vi "Spartan HTTP Error Reply.vi"(2 "message":string, 3 "status code":i32) -> (0 "content":string, 1 "header":string)   [LabVIEW 2011]
uses:
  Addons/internet/http/config.llb/HTTP SRM.vi
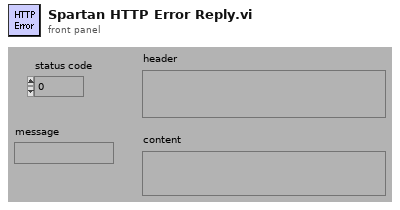
[diagram p1: front panel]
types:
  T1 = typedef "Keyed Array.ctl" = cluster{"keys":string[], "values":string[]}
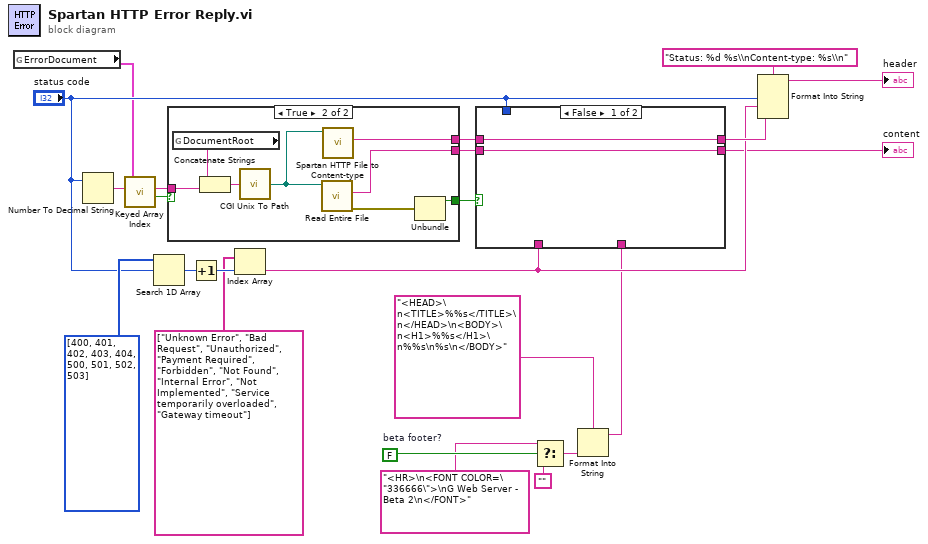
[diagram p0: block diagram]
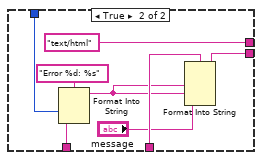
[diagram p2: hidden frame]
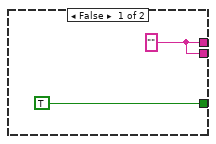
[diagram p3: hidden frame]
diagram:
  w5 = FALSE  # beta footer?
  n1 = global read "HTTP SRM.vi" "ErrorDocument"() -> (w1:T1)
  n2 = Number To Decimal String(number="status code") -> (decimal integer string=w18:string)  [unwired: 1 out]
  n3 = call "Keyed Array Index.vi"("key"=w18, "array in"=w1) -> ("valid key"=w17:bool, "value"=w16:string)  [unwired: 2 in, 2 out]
  n4 = Search 1D Array(1D array=i32[] [400, 401, 402, 403, 404, 500, 501, 502, 503], element="status code") -> (index of element=w22:i32)  [unwired: 1 out]
  n5 = case shown="True" w17 {
    tunnel: w16 -> [_ w31]
    tunnel: [TRUE ("status") w33] -> w15
    tunnel: [w24 w30] -> w14
    tunnel: [w24 w27] -> w13
    frame False {
      w24 = "" ("content type")
    }
    frame True {
      n6 = global read "HTTP SRM.vi" "DocumentRoot"() -> (w26:string)
      n7 = Concatenate Strings(w26, w31) -> (w32:string)
      n8 = call "CGI Unix To Path.vi"("unix path"=w32) -> ("platform path"=w29:path)  [unwired: 1 out]
      n9 = call "Read Entire File.vi"("path"=w29) -> ("error out"=w28:errorcluster, "data"=w27:string)  [unwired: 2 in, 7 out]
      n10 = call "Spartan HTTP File to Content-type.vi"("file path"=w29) -> ("content-type"=w30:string)  [unwired: 3 in, 7 out]
      n11 = Unbundle(w28) -> ("status"=w33:bool)  [unwired: 2 out]
    }
  }
  n12 = Increment(x=w22) -> (x+1=w23:i32)
  n13 = Index Array(array=string[] ["Unknown Error", "Bad Request", "Unauthorized", "Payment Required", "Forbidden", "Not Found", "Internal Error", "Not Implemented", "Service temporarily overloaded", "Gateway timeout"], index=w23) -> (element=w11:string)
  n14 = Select(t="<HR>\n<FONT COLOR=\"336666\">\nG Web Server - Beta 2\n</FONT>", s=w5, f="") -> (s? t:f=w3:string)
  n15 = Format Into String(format string="<HEAD>\n<TITLE>%%s</TITLE>\n</HEAD>\n<BODY>\n<H1>%%s</H1>\n%%s\n%s\n</BODY>", w3) -> (resulting string=w8:string)  [unwired: 2 in, 1 out]
  n16 = case shown="False" w15 {
    tunnel: w14 -> [w35 _]
    tunnel: [w35 "text/html"] -> w12
    tunnel: w13 -> [w34 _]
    tunnel: [w34 w37] -> w7
    tunnel: w11 -> [_ w41]
    tunnel: "status code" -> [_ w40]
    tunnel: w8 -> [_ w39]
    frame False {
    }
    frame True {
      n17 = Format Into String(format string="Error %d: %s", w40, w41) -> (resulting string=w38:string)  [unwired: 2 in, 1 out]
      n18 = Format Into String(format string=w39, w38, w38, "message") -> (resulting string=w37:string)  [unwired: 2 in, 1 out]
    }
  }
  "content" <- w7
  n19 = Format Into String(format string="Status: %d %s\\nContent-type: %s\\n", "status code", w11, w12) -> (resulting string=→"header":string)  [unwired: 2 in, 1 out]
